vi "CALCULATION FOR ACOUSTICS.vi"(8 "error in (no error)":errorcluster, 9 "ALPHA-INPUT":dbl[](array[numeric]), 10 "PRE-INPUT":dbl[](array[numeric]), 11 "INPUT":dbl[](array[numeric])) -> (0 "error out":errorcluster, 3 "0UTPUT":dbl[](array[numeric]))   [LabVIEW 2025]
panel:
  out "ALPHA-INPUT 2":dbl[](array[numeric])
  out "PRE-INPUT 2":dbl[](array[numeric])
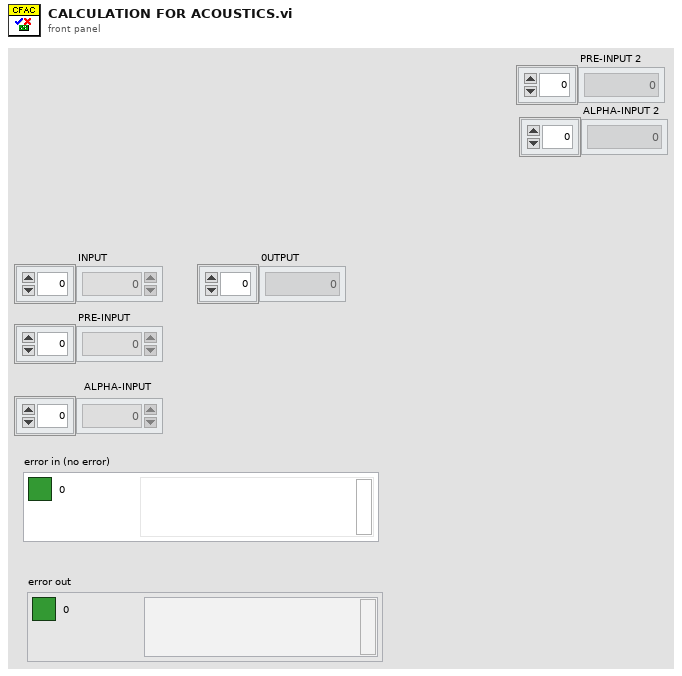
[diagram p1: front panel]
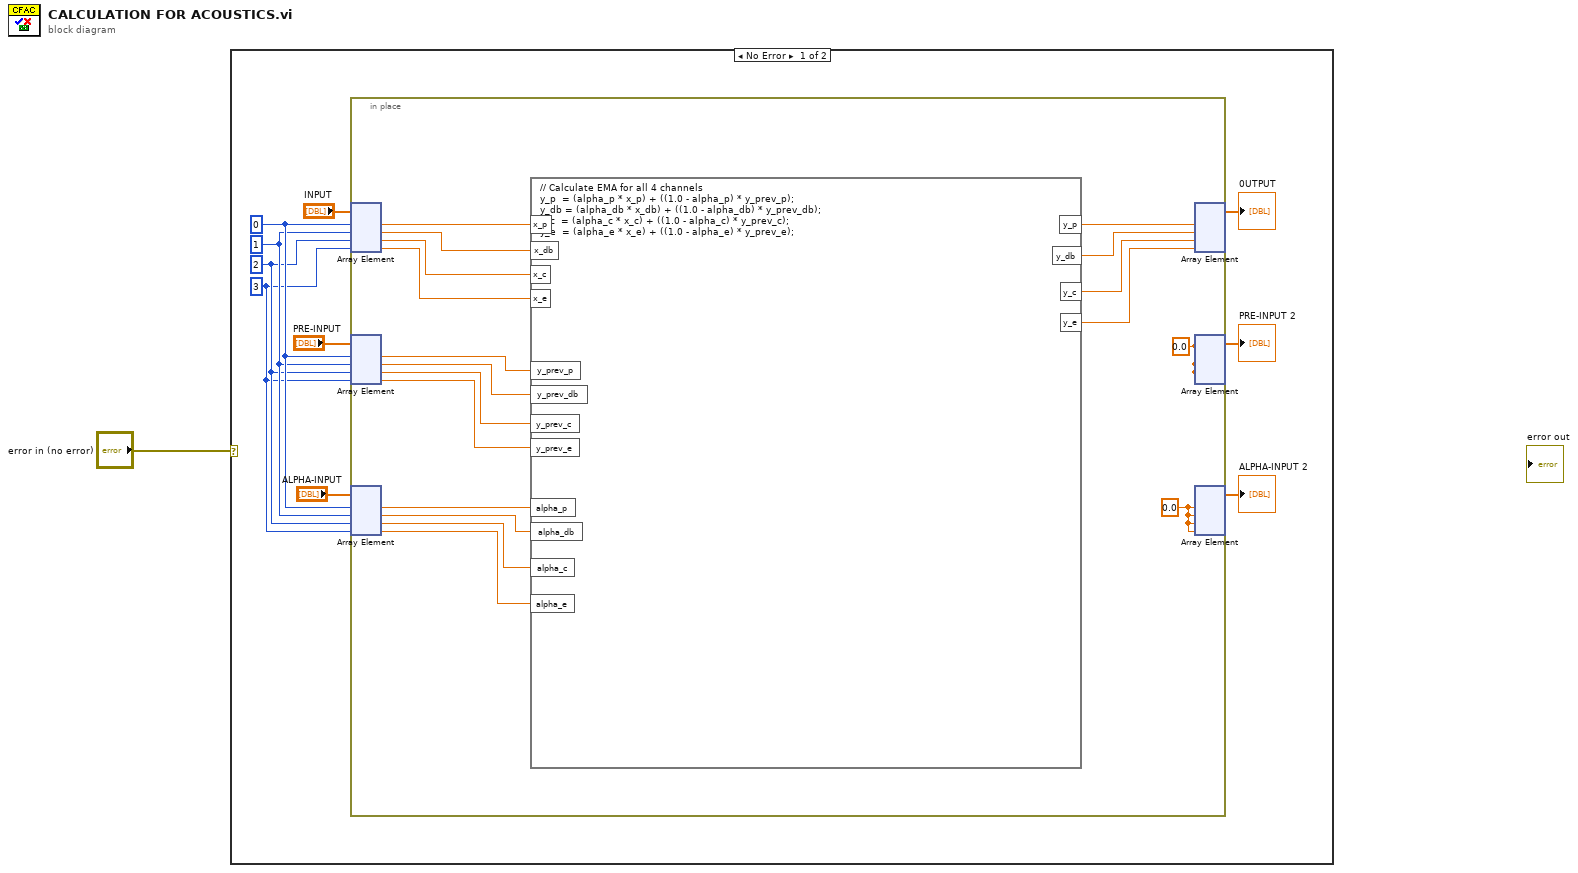
[diagram p0: block diagram]
diagram:
  n1 = case shown="No Error" "error in (no error)" {
    frame No Error {
      w5 = 3
      w6 = 2
      w7 = 1
      w8 = 0
      n2 = in-place {
        w12 = 0.0 ("element")
        w13 = 0.0 ("element")
        n3 = in-place-array #1("INPUT", w8, w7, w6, w5) -> (w29:dbl, w28:dbl, w27:dbl, w26:dbl)
        n4 = in-place-array #2("PRE-INPUT", w8, w7, w6, w5) -> (w25:dbl, w24:dbl, w23:dbl, w22:dbl)
        n5 = in-place-array #3("ALPHA-INPUT", w8, w7, w6, w5) -> (w21:dbl, w20:dbl, w19:dbl, w18:dbl)
        n6 = formula code="// Calculate EMA for all 4 channels\ny_p  = (alpha_p * x_p) + ((1.0 - alpha_p) * y_prev_p);\ny_db = (alpha_db * x_db) + ((1.0 - alpha_db) * y_prev_db);\ny_c  = (alpha_c * x_c) + ((1.0 - alpha_c) * y_prev_c);\ny_e  = (alpha_e * x_e) + ((1.0 - alpha_e) * y_prev_e);"("alpha_p"=w21, "x_p"=w29, "y_prev_p"=w25, "alpha_db"=w20, "x_db"=w28, "y_prev_db"=w24, "alpha_c"=w19, "x_c"=w27, "y_prev_c"=w23, "alpha_e"=w18, "x_e"=w26, "y_prev_e"=w22) -> ("y_p"=w17:dbl, "y_db"=w16:dbl, "y_c"=w15:dbl, "y_e"=w14:dbl)
        n7 = in-place-array #1(w17, w16, w15, w14) -> (→"0UTPUT":dbl[])  [unwired: 4 out]
        n8 = in-place-array #2(w13, w13, w13, w13) -> (→"PRE-INPUT 2":dbl[])  [unwired: 4 out]
        n9 = in-place-array #3(w12, w12, w12, w12) -> (→"ALPHA-INPUT 2":dbl[])  [unwired: 4 out]
      }
    }
    frame Error {
    }
  }
